vi "CRYAppend Sequence Folder Name in Titlebar.vi"   [LabVIEW 2013]
uses:
  CRYProject/CRYProject Editor Global.vi
  CRYMain Sub Window Global.vi
types:
  T1 = typedef "CRYTS.ctl" = cluster{"No.TS":u16, "TS File Path":path, "TS Name":string, "EditStepName":string, "Steps":T2[], "New State":bool, "Change State":bool, "Flattened CurveLib Data":string, "Document Data":string, "EditStepNo":u16, "Operator Start File":string, "Sequence Type":string, "Sequence Language":string}
  T2 = typedef "CRYStep.ctl" = cluster{"No.VI":i32, "Category":string, "StepName":string, "Seq setup flattened":string, "Comment":string, "Steps config.":bool[], "Jump config":i32[], "Start":dbl, "Increment":dbl, "Name":string, "Unit":string, "Y data":u16, "Y prefix":string, "Y dB ref":dbl, "Y unit":string, "Repeat State Array":cluster{"Start":dbl, "Increment":dbl, "Count":i32, "Num":i32}[]}
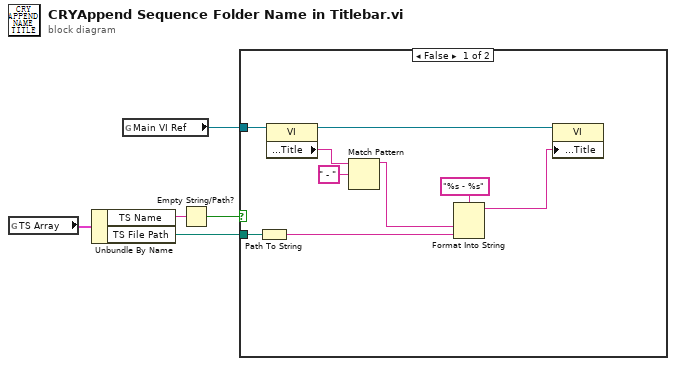
[diagram p0: block diagram]
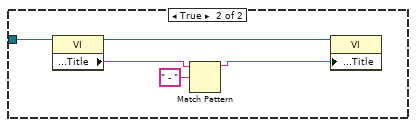
[diagram p2: hidden frame]
diagram:
  n1 = global read "CRYProject Editor Global.vi" "TS Array"() -> (w5:T1)
  n2 = Unbundle By Name(w5) -> ("TS Name"=w3:string, "TS File Path"=w1:path)
  n3 = global read "CRYMain Sub Window Global.vi" "Main VI Ref"() -> (w4:refnum<vi>)
  n4 = Empty String/Path?(string/path=w3) -> (empty?=w2:bool)
  n5 = case shown="False" w2 {
    tunnel: w4 -> [w14 w16]
    tunnel: w1 -> [w12 _]
    frame False {
      n6 = Path To String(path=w12) -> (string=w10:string)
      n7 = property class="VI"(reference=w14) -> (reference out=w13:refnum<vi>, "Front Panel.Title"=w8:string)  [unwired: 1 in, 1 out]
      n8 = Match Pattern(string=w8, regular expression=" - ") -> (before substring=w6:string)  [unwired: 1 in, 3 out]
      n9 = Format Into String(format string="%s - %s", w6, w10) -> (resulting string=w9:string)  [unwired: 2 in, 1 out]
      n10 = property class="VI"(reference=w13, "Front Panel.Title"=w9) -> ()  [unwired: 1 in, 2 out]
    }
    frame True {
      n11 = property class="VI"(reference=w16) -> (reference out=w19:refnum<vi>, "Front Panel.Title"=w18:string)  [unwired: 1 in, 1 out]
      n12 = Match Pattern(string=w18, regular expression=" - ") -> (before substring=w15:string)  [unwired: 1 in, 3 out]
      n13 = property class="VI"(reference=w19, "Front Panel.Title"=w15) -> ()  [unwired: 1 in, 2 out]
    }
  }
